vi "GotoZero.vi"(8 "Error In":errorcluster, 11 "AutoData":T1) -> (0 "Error Out":errorcluster, 3 "AutoData out":T1)   [LabVIEW 2019, in "AutoMode.lvlib"]
uses:
  AutoMode.lvlib
  Cluster - AutoModeData.ctl
  MainController/Cluster - TestSettings.ctl
  MainController/Cluster - HardwareConfiguration.ctl
  MainController/Cluster - TestResults.ctl
  Cluster - AutoModeMessage.ctl
  Enum - AutoModeState.ctl
  MainController/Cluster - MainControllerMessage.ctl
  MainController/Enum - MainState.ctl
  Mark10 API/WriteSpeed.vi
  Mark10 API/WriteCWTravelLimit.vi
  Mark10 API/Mark 10 TSTM-DC.lvlib
  EventLogger/EventLogger.lvlib
  MainController/MainController.lvlib
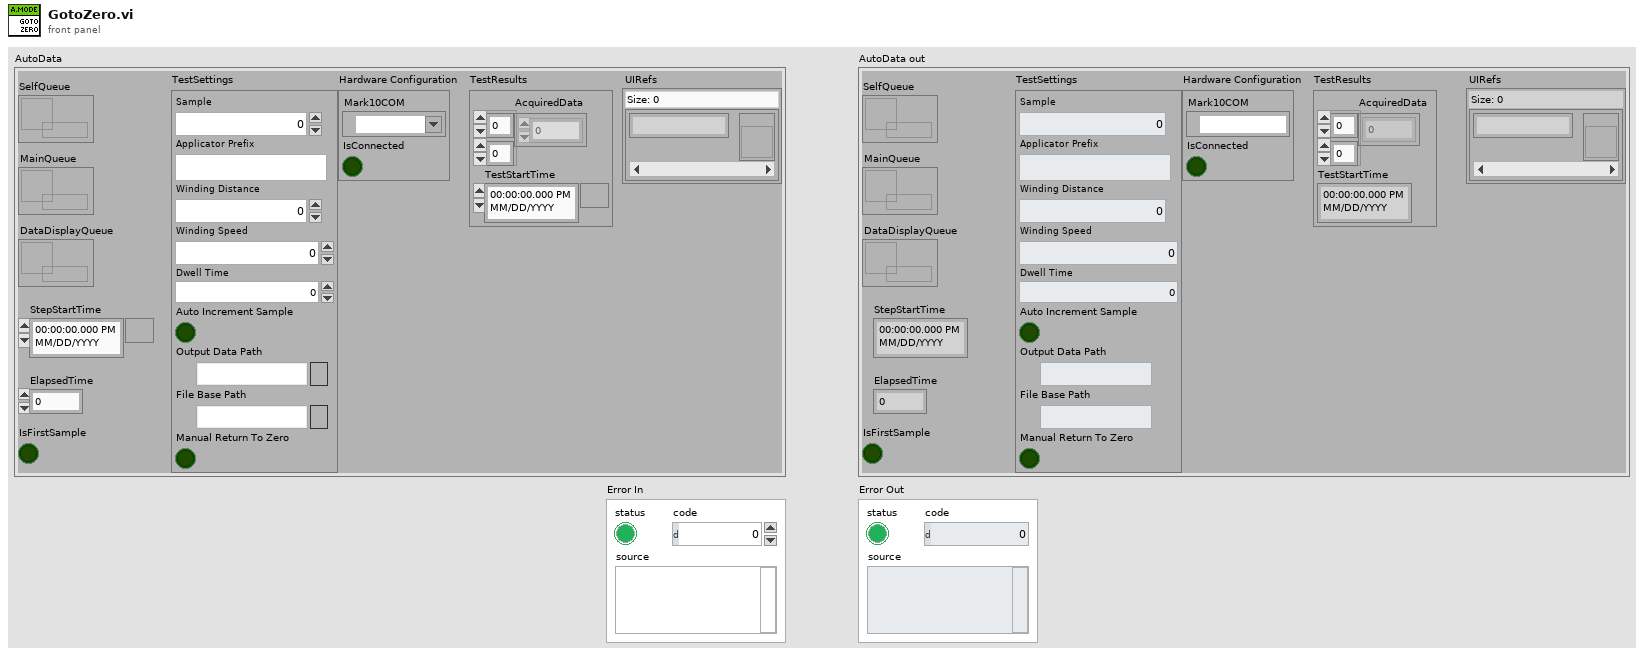
[diagram p1: front panel]
types:
  T1 = typedef "AutoMode.lvlib/Cluster - AutoModeData.ctl" = cluster{"DataDisplayQueue":refnum<queue>, "StepStartTime":timestamp, "TestSettings":T2, "Hardware Configuration":T3, "TestResults":T4, "ElapsedTime":dbl, "IsFirstSample":bool, "SelfQueue":refnum<queue>, "MainQueue":refnum<queue>, "UIRefs":map{string, refnum<vi>}}
  T2 = typedef "MainController.lvlib/Cluster - TestSettings.ctl" = cluster{"Sample":u32, "Applicator Prefix":string, "Winding Distance":dbl, "Winding Speed":dbl, "Dwell Time":dbl, "Auto Increment Sample":bool, "Output Data Path":path, "File Base Path":path, "Manual Return To Zero":bool}
  T3 = typedef "MainController.lvlib/Cluster - HardwareConfiguration.ctl" = cluster{"Mark10COM":refnum<visa-resource-name>, "IsConnected":bool}
  T4 = typedef "MainController.lvlib/Cluster - TestResults.ctl" = cluster{"AcquiredData":dbl[][], "TestStartTime":timestamp}
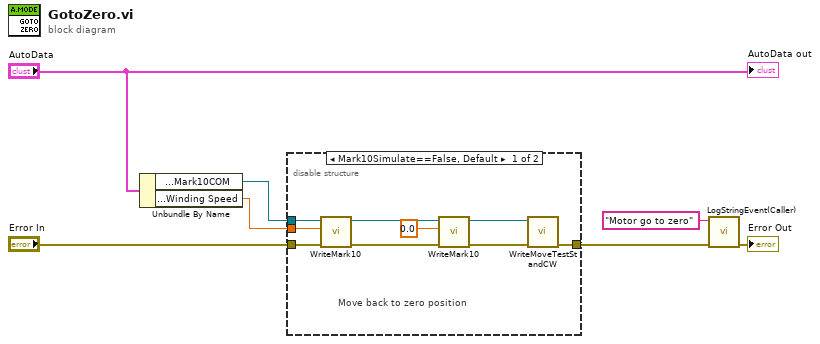
[diagram p0: block diagram]
diagram:
  n1 = Unbundle By Name("AutoData") -> ("Hardware Configuration.Mark10COM"=w4:refnum<visa-resource-name>, "TestSettings.Winding Speed"=w5:dbl)
  n2 = disable-structure shown="Mark10Simulate==False, Default" {
    disable-tunnel: [w15 w17] -> w6
    disable-tunnel: w5 -> [w12 _]
    disable-tunnel: w4 -> [w11 _]
    disable-tunnel: "Error In" -> [w9 w17]
    frame condition #0 (active) {
      # "Move back to zero position"
      n3 = call-poly "WriteMark10.vi"("error in"=w9, "Speed"=w12, "VISA resource name"=w11) -> ("error out"=w8:errorcluster, "VISA resource name out"=w10:refnum<visa-resource-name>)  [unwired: 7 in]
      n4 = call-poly "WriteMark10.vi"("error in"=w8, "CWTravelLimit"=0.0, "VISA resource name"=w10) -> ("error out"=w16:errorcluster, "VISA resource name out"=w14:refnum<visa-resource-name>)  [unwired: 7 in]
      n5 = call "WriteMoveTestStandCW.vi"("error in"=w16, "VISA resource name"=w14) -> ("error out"=w15:errorcluster)  [unwired: 8 in, 1 out]
    }
    frame condition #1 {
    }
  }
  n6 = call "LogStringEvent(Caller).vi"("Error In"=w6, "Field"="Motor go to zero") -> ("Error Out"=→"Error Out":errorcluster)  [unwired: 9 in]
  "AutoData out" <- "AutoData"
